vi "PerfAddRemove.vi"() -> (3 "Add time":dbl format="%.2p")   [LabVIEW 2024, in "CircularBuffer.Test.Perf.lvlib"]
uses:
  CircularBuffer.Test.Perf.lvlib
  <vilib>/Analysis/NI_AALBase.lvlib
  <vilib>/Analysis/baseanly.llb/Mean (DBL).vi
  bbc7a370-0dd1-4504-b3b0-06d700688abf.vi
  dcabc875-db76-4c53-9c4f-cf505999d426.vi
  6045e48b-d2eb-4048-91f0-a5fde5ba3311.vi
  10666d2b-b659-4efd-8cbe-8400d97b5c3b.vi
panel:
  out "remove time":dbl format="%.2p"
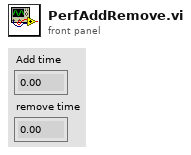
[diagram p1: front panel]
types:
  T1 = cluster{"buffer":u32[], "head":i32, "tail":i32, "size":i32, "capacity":i32}
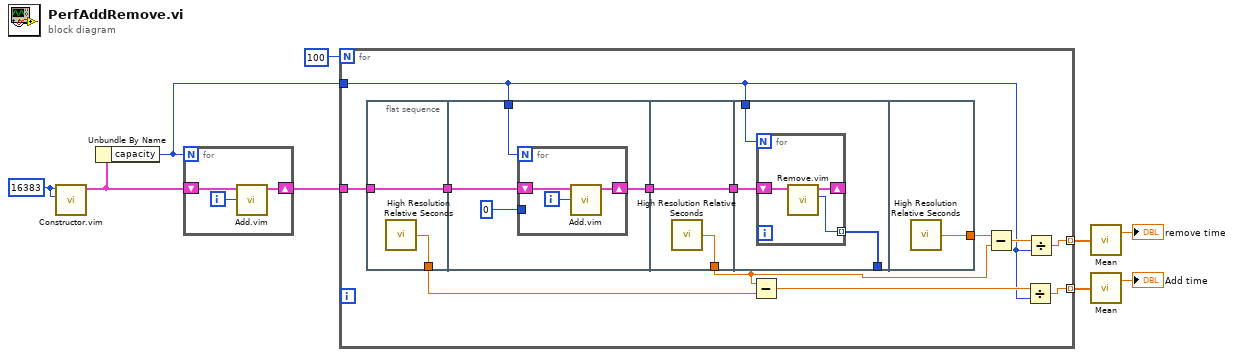
[diagram p0: block diagram]
diagram:
  w4 = u32 16383 ("Capacity")
  n1 = call "Constructor.vim"("Capacity"=w4, "Placeholder Type"=w4) -> ("CircularBuffer out"=w2:T1)  [unwired: 9 in]
  n2 = Unbundle By Name(w2) -> ("capacity"=w1:i32)
  n3 = for {
    N: w1 -> [_]
    shift-right: [w11] -> w3
    shift-left: w2 -> [w12]
    i -> [w10]
    n4 = call "Add.vim"("New Element"=w10, "CircularBuffer in"=w12) -> ("CircularBuffer out"=w11:T1)  [unwired: 7 in, 2 out]
  }
  n5 = for {
    N: 100 -> [_]
    tunnel: [w16] -> w9 mode=indexing
    tunnel: w3 -> [w23]
    tunnel: [w14] -> w5 mode=indexing
    tunnel: w1 -> [w13]
    n6 = flat-sequence {
      tunnel: w23 -> [w26]
      tunnel: [w26] -> w20
      tunnel: [w25] -> w18
      tunnel: [w29] -> w21
      tunnel: w20 -> [w30]
      tunnel: w13 -> [w27]
      tunnel: [w35] -> w19
      tunnel: [w34] -> w22
      tunnel: w21 -> [w34]
      tunnel: [w38] -> _
      tunnel: w22 -> [w37]
      tunnel: w13 -> [w36]
      tunnel: [w42] -> w24
      frame #0 {
        n7 = call <vilib>:"High Resolution Relative Seconds.vi"() -> ("relative seconds"=w25:dbl)
      }
      frame #1 {
        n8 = for {
          N: w27 -> [_]
          shift-right: [w32] -> w29
          shift-left: w30 -> [w33]
          tunnel: u32 0 ("Capacity") -> [_]
          i -> [w31]
          n9 = call "Add.vim"("New Element"=w31, "CircularBuffer in"=w33) -> ("CircularBuffer out"=w32:T1)  [unwired: 7 in, 2 out]
        }
      }
      frame #2 {
        n10 = call <vilib>:"High Resolution Relative Seconds.vi"() -> ("relative seconds"=w35:dbl)
      }
      frame #3 {
        n11 = for {
          N: w36 -> [_]
          shift-right: [w39] -> _
          shift-left: w37 -> [w41]
          tunnel: [w40] -> w38 mode=indexing
          n12 = call "Remove.vim"("CircularBuffer in"=w41) -> ("Element"=w40:u32, "CircularBuffer out"=w39:T1)  [unwired: 8 in, 1 out]
        }
      }
      frame #4 {
        n13 = call <vilib>:"High Resolution Relative Seconds.vi"() -> ("relative seconds"=w42:dbl)
      }
    }
    n14 = Subtract(x=w19, y=w18) -> (x-y=w15:dbl)
    n15 = Subtract(x=w24, y=w19) -> (x-y=w17:dbl)
    n16 = Divide(x=w15, y=w13) -> (x/y=w14:dbl)
    n17 = Divide(x=w17, y=w13) -> (x/y=w16:dbl)
  }
  n18 = call-poly <vilib>:"Mean.vi"("X"=w9) -> ("mean"=→"remove time":dbl)  [unwired: 1 out]
  n19 = call-poly <vilib>:"Mean.vi"("X"=w5) -> ("mean"=→"Add time":dbl)  [unwired: 1 out]
